vi "_019.vi"() -> ()   [LabVIEW 2024]
panel:
  out "all upper case string":string
  in  "string":string
  out "all lower case string":string
  in  "string":string
  out "result string":string
  out "replaced substring":string
  in  "offset (0)":i32
  in  "length (len. of substring)":i32
  in  "substring (\"\")":string
  in  "string":string
  # "String functions :"
  # "(Basics)"
  # "Replace Substring :"
  # "Upper case to Lower case :"
  # "Lower case to Upper case :"
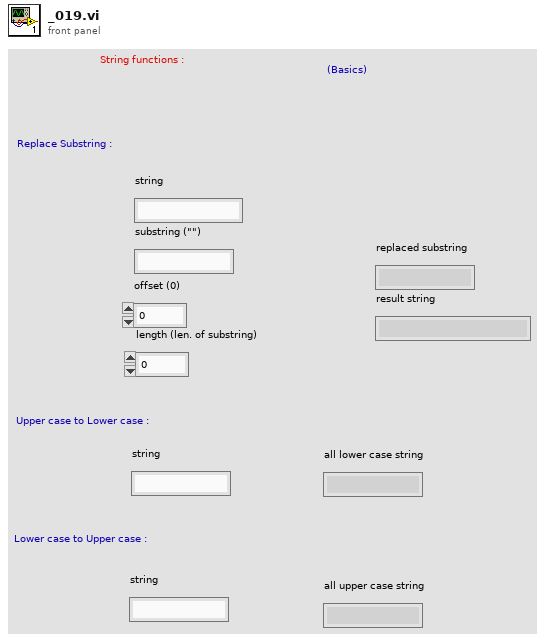
[diagram p1: front panel]
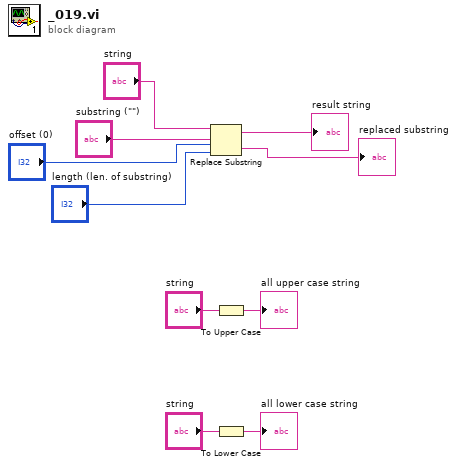
[diagram p0: block diagram]
diagram:
  n1 = Replace Substring(2:"length (len. of substring)", 3:"offset (0)", 4:"substring (\"\")", 5:"string") -> (0:→"replaced substring":string, 1:→"result string":string)
  n2 = To Upper Case(1:"string") -> (0:→"all upper case string":string)
  n3 = To Lower Case(string="string") -> (all lower case string=→"all lower case string":string)
